vi "FullOn.vi"(8 "error in (no error)":errorcluster, 11 "DCMotor in":refnum<class "DCMotor.lvclass">) -> (0 "error out":errorcluster, 3 "DCMotor out":refnum<class "DCMotor.lvclass">)   [LabVIEW 2022 SP3, in "Motorshield.lvlib" / "DCMotor.lvclass"]
uses:
  DCMotor.lvclass
  DCMotor.lvclass/DCMotor.ctl
  Motorshield/Motorshield.lvclass
  C:/Users/Carlos/Desktop/onlab/source/Motorshield/Motorshield/Motorshield.lvclass
  C:/Users/Carlos/Desktop/onlab/source/Motorshield/DCMotor/DCMotor.lvclass
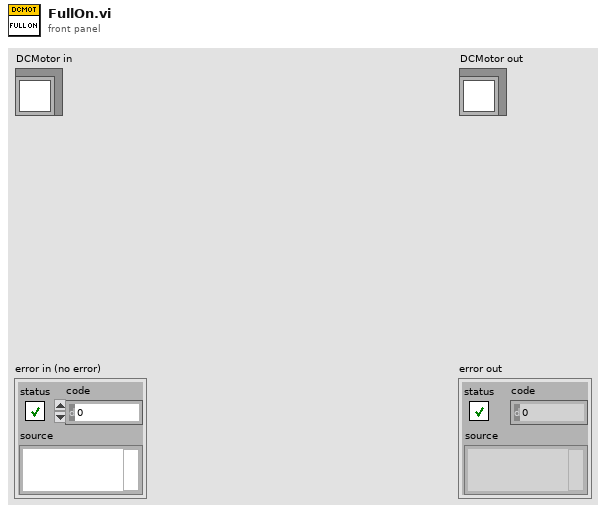
[diagram p1: front panel]
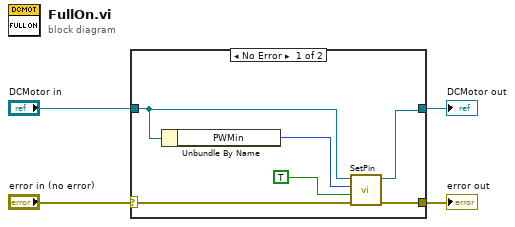
[diagram p0: block diagram]
diagram:
  n1 = case shown="No Error" "error in (no error)" {
    selector: "error in (no error)" -> [w7 w12]
    tunnel: [w8 w12] -> w3
    tunnel: [w5 w11] -> w1
    tunnel: "DCMotor in" -> [w6 w11]
    frame No Error {
      n2 = Unbundle By Name(w6) -> ("PWMin"=w10:u8)
      n3 = call "SetPin.vi"("error in (no error)"=w7, "Value"=TRUE, "Led num"=w10, "Motorshield in"=w6) -> ("error out"=w8:errorcluster, "Motorshield out"=w5:refnum<class "DCMotor.lvclass">)  [unwired: 6 in]
    }
    frame Error {
    }
  }
  "error out" <- w3
  "DCMotor out" <- w1
